vi "init.vi"(8 "error in (no error)":errorcluster, 10 "Resource":string, 11 "DmmKeysight in":refnum<class "DmmKeysight.lvclass">) -> (0 "error out":errorcluster, 3 "DmmKeysight out":refnum<class "DmmKeysight.lvclass">)   [LabVIEW 2023, in "DmmKeysight.lvclass"]
doc: "<b>Author:</b> Wolfgang\n<b>Description:</b> Method to initialize an instrument by resource name (defined in NI MAX) for any instrument category."
uses:
  DmmKeysight.lvclass
  Driver/TypeDef/configuration.ctl
  Driver/TypeDef/mode.ctl
  DmmKeysight.lvclass/DmmKeysight.ctl
  Multimeter.lvclass
  Driver/Keysight-34450A.lvlib
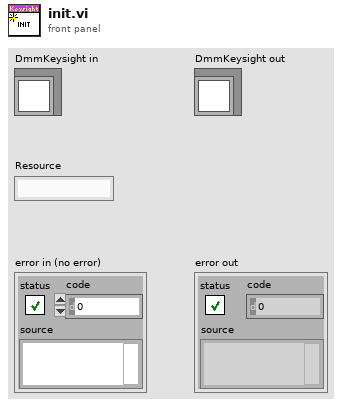
[diagram p1: front panel]
types:
  T1 = typedef "Keysight-34450A.lvlib/configuration.ctl" = cluster{"mode":T2, "Range":dbl, "Resolution":dbl}
  T2 = typedef "Keysight-34450A.lvlib/mode.ctl" = enum16{"DC_Voltage", "AC_Voltage", "DC_Current", "AC_Current", "Resistance"}
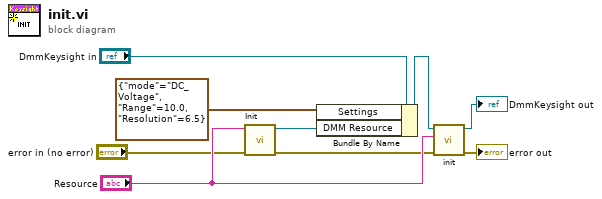
[diagram p0: block diagram]
diagram:
  n1 = call "Init.vi"("error in (no error)"="error in (no error)", "VISA resource name"="Resource") -> ("error out"=w4:errorcluster, "VISA resource name out"=w2:refnum<visa-resource-name>)  [unwired: 7 in, 1 out]
  n2 = Bundle By Name(cluster="DmmKeysight in", "Settings"=T1 {"mode"=enum."DC_Voltage", "Range"=10.0, "Resolution"=6.5}, "DMM Resource"=w2) -> (w3:refnum<class "DmmKeysight.lvclass">)
  n3 = call-parent "init.vi"("error in (no error)"=w4, "Resource"="Resource", "Instrument in"=w3) -> ("error out"=→"error out":errorcluster, "Instrument out"=→"DmmKeysight out":refnum<class "DmmKeysight.lvclass">)  [unwired: 7 in]
